vi "update voltage outputs.vi"(9 "Message handler data":T1, 11 "Data":variant) -> (0 "error out":errorcluster)   [LabVIEW 2018]
uses:
  Type Defs/Message loop data.ctl
  Type Defs/FPGA reference.ctl
  Type Defs/RT Status.ctl
  <vilib>/Utility/error.llb/Error Cluster From Error Code.vi
  <vilib>/rvi/errors/niLvFpgaAdjustHostInterfaceError.vi
  <vilib>/rvi/interface/nirviReadWriteControl/nirviReadWriteControl.xnode
  FPGA Bitfiles/CompressorRigV2_CompressorFPGA_FPGAMainV3_7sPRekuravM.lvbitx
  NiFpgaLv.dll
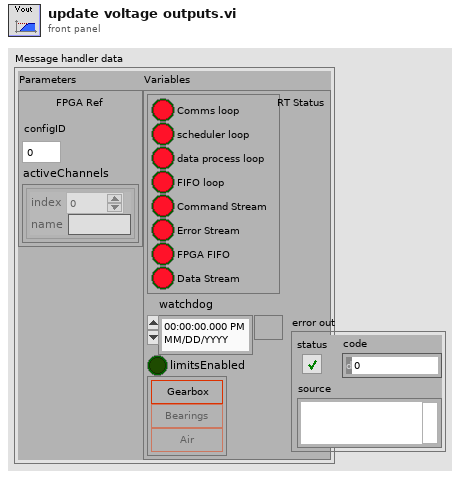
[diagram p1: front panel]
types:
  T1 = typedef "Message loop data.ctl" = cluster{"Parameters":cluster{"FPGA Ref":T2, "configID":u32, "activeChannels":cluster{"index":u16, "name":string}[]}, "Variables":cluster{"RT Status":T3, "watchdog":timestamp, "limitsEnabled":bool, "Interlocks":cluster{"gearboxOil":bool, "bearingOil":bool, "gearboxAir":bool}}}
  T2 = typedef "FPGA reference.ctl" = refnum<k20>
  T3 = typedef "RT Status.ctl" = cluster{"Comms loop":bool, "scheduler loop":bool, "data process loop":bool, "FIFO loop":bool, "Command Stream":bool, "Error Stream":bool, "FPGA FIFO":bool, "Data Stream":bool}
  T4 = cluster{"channel":i32, "output Value":fxp<+/-,20,5>}
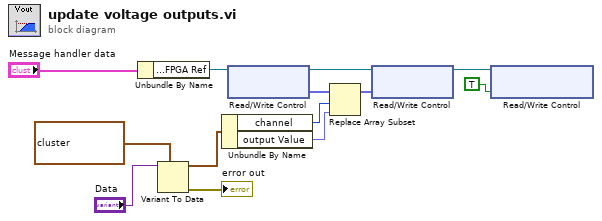
[diagram p0: block diagram]
diagram:
  n1 = Unbundle By Name("Message handler data") -> ("Parameters.FPGA Ref"=w12:T2)
  n2 = Variant To Data(type=T4 {"channel"=0, "output Value"=0.0}, Variant="Data") -> (data=w7:T4, error out=→"error out":errorcluster)  [unwired: 1 in]
  n3 = Unbundle By Name(w7) -> ("channel"=w5:i32, "output Value"=w4:fxp<+/-,20,5>)
  n4 = xnode "Read/Write Control"("FPGA VI Reference In"=w12) -> ("FPGA VI Reference Out"=w11:T2, "Voltage Out"=w10:fxp<+/-,20,5>[])  [unwired: 1 in, 1 out]
  n5 = Replace Array Subset(array=w10, new element=w4, index=w5) -> (w6:fxp<+/-,20,5>[])
  n6 = xnode "Read/Write Control"("FPGA VI Reference In"=w11, "Voltage Out"=w6) -> ("FPGA VI Reference Out"=w3:T2)  [unwired: 1 in, 1 out]
  n7 = xnode "Read/Write Control"("FPGA VI Reference In"=w3, "Update Outputs"=TRUE ("Enable Data FIFO")) -> ()  [unwired: 1 in, 2 out]
